vi "PXI-General Init.vi"(7 "Double Buffer Mode":enum32{"OFF", "ENABLED", "FORCED"}(ring)=enum."ENABLED", 8 "error in (no error)":errorcluster) -> (0 "error out":errorcluster)   [LabVIEW 2020]
doc: "Performs common PXI DAQ initialization tasks. Simplifies configuration process in higher-level measurement VIs."
uses:
  Type Defs/PXI-AI Transfer Mode.ctl
  Type Defs/PXI-DO Signal Bank Action.ctl
  DAQ Engine VIs/PXI Globals.vi
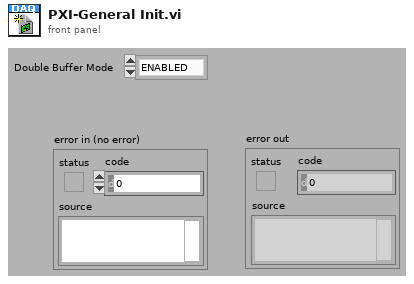
[diagram p1: front panel]
types:
  T1 = typedef "PXI-DO Signal Bank Action.ctl" = enum16{"Clear", "Write", "Read"}
  T2 = typedef "PXI-AI Transfer Mode.ctl" = enum16{"Queue", "Data Bank", "No Transfer"}
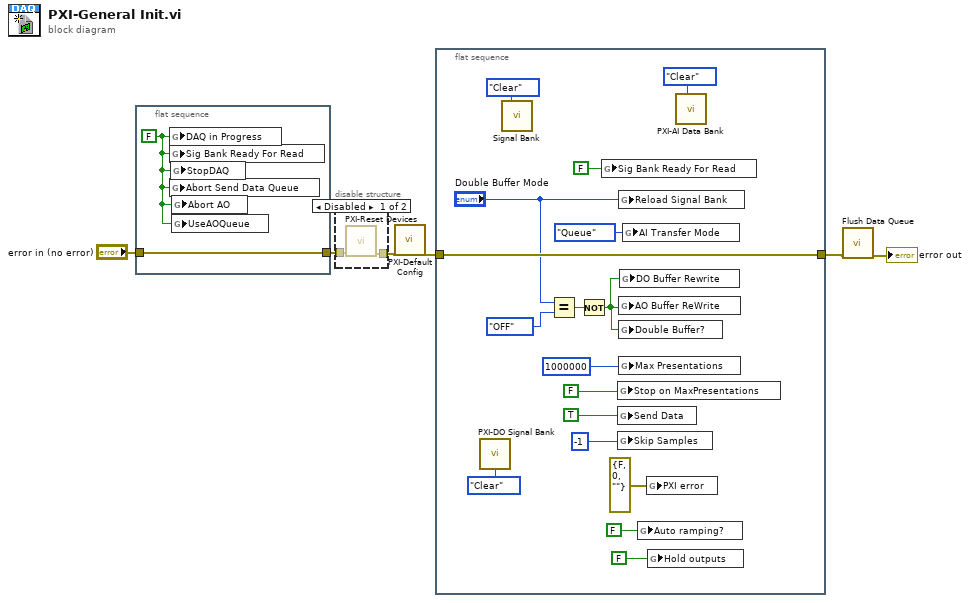
[diagram p0: block diagram]
diagram:
  n1 = flat-sequence {
    tunnel: "error in (no error)" -> [w8]
    tunnel: [w8] -> w5
    frame #0 {
      w7 = FALSE ("DAQ in Progress")
      n2 = global write "PXI Globals.vi" "DAQ in Progress"(w7) -> ()
      n3 = global write "PXI Globals.vi" "Sig Bank Ready For Read"(w7) -> ()
      n4 = global write "PXI Globals.vi" "Abort Send Data Queue"(w7) -> ()
      n5 = global write "PXI Globals.vi" "StopDAQ"(w7) -> ()
      n6 = global write "PXI Globals.vi" "Abort AO"(w7) -> ()
      n7 = global write "PXI Globals.vi" "UseAOQueue"(w7) -> ()
    }
  }
  n8 = disable-structure shown="Disabled" {
    disable-tunnel: w5 -> [w10 w11]
    disable-tunnel: [w9 w11] -> w4
    frame Disabled {
      n9 = call "PXI-Reset Devices.vi"("error in"=w10) -> ("error out"=w9:errorcluster)  [unwired: 10 in]
    }
    frame Enabled {
    }
  }
  n10 = call "PXI-Default Config.vi"("error in (no error)"=w4) -> ("error out"=w2:errorcluster)  [unwired: 26 in]
  n11 = flat-sequence {
    tunnel: w2 -> [w24]
    tunnel: [w24] -> w1
    frame #0 {
      n12 = call "PXI-DO Signal Bank.vi"("Action"=PXI-DO_Signal_Bank_Action."Clear") -> ()  [unwired: 13 in, 2 out]
      n13 = call "Signal Bank.vi"("Action"=enum16{"Add", "Replace ID", "Read ID", "Clear"}."Clear") -> ()  [unwired: 13 in, 2 out]
      n14 = Equal?(x="Double Buffer Mode", y=enum32{"OFF", "ENABLED", "FORCED"}."OFF" ("Reload Signal Bank")) -> (x = y?=w21:bool)
      n15 = Not(x=w21) -> (.not. x?=w16:bool)
      n16 = global write "PXI Globals.vi" "Sig Bank Ready For Read"(FALSE ("Sig Bank Ready For Read")) -> ()
      n17 = global write "PXI Globals.vi" "Stop on MaxPresentations"(FALSE ("Stop on MaxPresentations")) -> ()
      n18 = global write "PXI Globals.vi" "Send Data"(TRUE ("Stop on MaxPresentations")) -> ()
      n19 = global write "PXI Globals.vi" "Skip Samples"(-1 ("Skip Samples")) -> ()
      n20 = global write "PXI Globals.vi" "Reload Signal Bank"("Double Buffer Mode") -> ()
      n21 = global write "PXI Globals.vi" "AO Buffer ReWrite"(w16) -> ()
      n22 = global write "PXI Globals.vi" "Double Buffer?"(w16) -> ()
      n23 = global write "PXI Globals.vi" "Max Presentations"(1000000 ("MaxPresentations")) -> ()
      n24 = global write "PXI Globals.vi" "DO Buffer Rewrite"(w16) -> ()
      n25 = global write "PXI Globals.vi" "AI Transfer Mode"(PXI-AI_Transfer_Mode."Queue" ("AI Transfer Mode")) -> ()
      n26 = global write "PXI Globals.vi" "Auto ramping?"(FALSE ("Auto ramping?")) -> ()
      n27 = global write "PXI Globals.vi" "PXI error"(errorcluster {"status"=FALSE, "code"=0, "source"=""} ("PXI error")) -> ()
      n28 = global write "PXI Globals.vi" "Hold outputs"(FALSE ("Auto ramping?")) -> ()
      n29 = call "PXI-AI Data Bank.vi"("Action"=PXI-DO_Signal_Bank_Action."Clear") -> ()  [unwired: 9 in, 2 out]
    }
  }
  n30 = call "Flush Data Queue.vi"("error in (no error)"=w1) -> ("error out"=→"error out":errorcluster)  [unwired: 10 in]
